vi "BasicAppPath.vi"(8 "错误输入（无错误）":errorcluster) -> (0 "error out":errorcluster, 3 "AppPath":path)   [LabVIEW 2015]
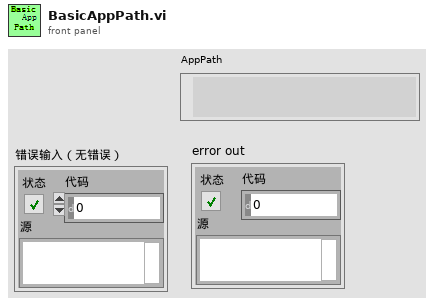
[diagram p1: front panel]
types:
  T1 = enum32{"invalid app kind", "Development System", "Run Time System", "Student Edition", "Embedded LabVIEW", "Evaluation", "Custom"}
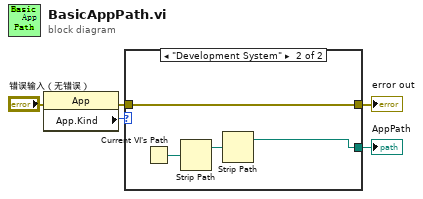
[diagram p0: block diagram]
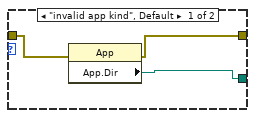
[diagram p2: hidden frame]
diagram:
  n1 = property class="App"(error in="错误输入（无错误）") -> (error out=w2:errorcluster, "App.Kind"=w5:T1)  [unwired: 1 in, 1 out]
  n2 = case shown="\"Development System\"" w5 {
    tunnel: [w6 w9] -> w4
    tunnel: w2 -> [w8 w10]
    tunnel: [w7 w10] -> w1
    frame "invalid app kind", Default {
      n3 = property class="App"(error in=w8) -> (error out=w7:errorcluster, "App.Dir"=w6:path)  [unwired: 1 in, 1 out]
    }
    frame "Development System" {
      n4 = Current VI's Path() -> (path=w12:path)
      n5 = Strip Path(path=w12) -> (stripped path=w11:path)  [unwired: 1 out]
      n6 = Strip Path(path=w11) -> (stripped path=w9:path)  [unwired: 1 out]
    }
  }
  "AppPath" <- w4
  "error out" <- w1
